vi "探头窗口-32-4列.vi"() -> ()   [LabVIEW 2017]
panel:
  in  "更新数据":T1
  in  "停止信号":bool=TRUE
  out "更新数据？":bool=TRUE
  out "引用-切回列表模式？":refnum<vi>
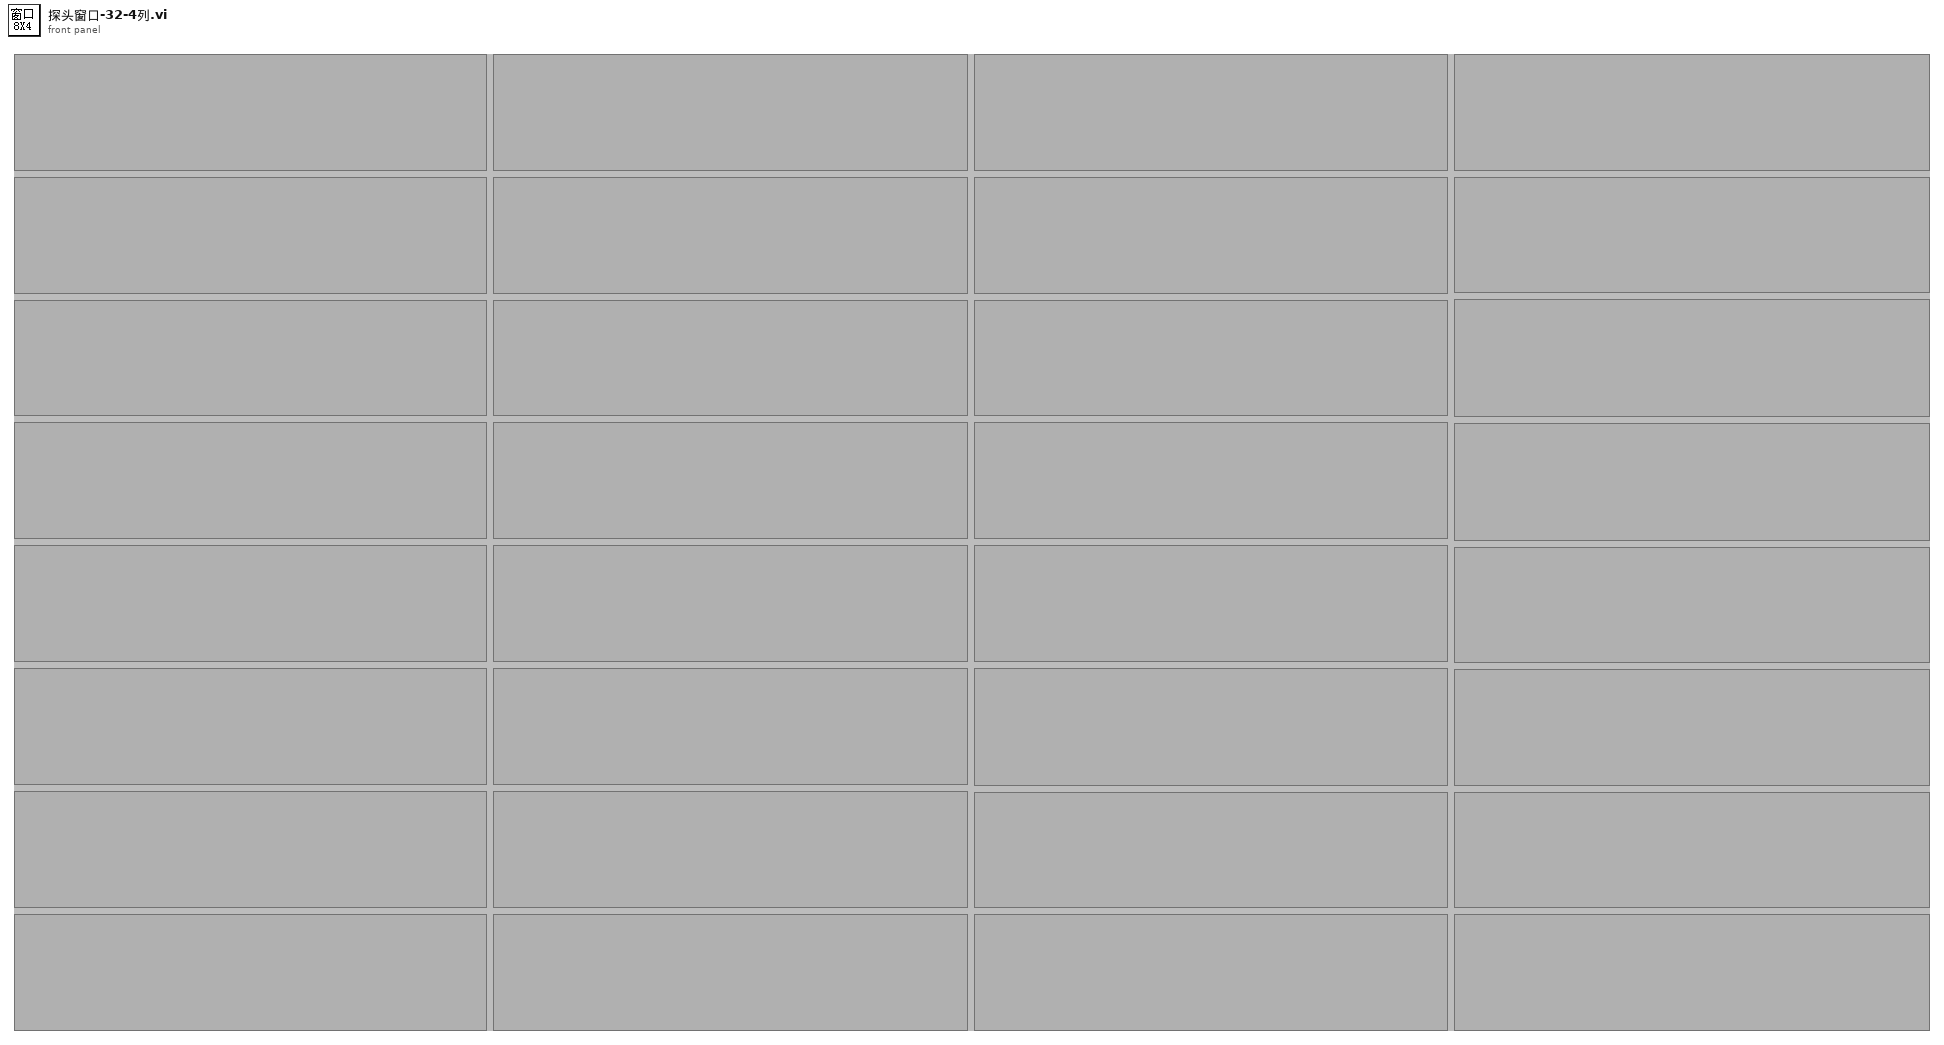
[diagram p1: front panel]
types:
  T1 = cluster{"探头启用状态？":bool[], "测量值":cluster{"X":timestamp, "Y":dbl}[], "限值":cluster{"限值1":dbl, "限值2":dbl, "探头限值":enum16{"一级限值", "二级限值"}}[], "报警状态":enum16{"正常", "一级报警", "二级报警", "累积报警"}[], "探头信息":string[], "累积剂量":cluster{"设备名称":string, "启用累积？":bool, "起始时间":timestamp, "累积剂量":dbl, "累积报警阈值":dbl}[]}
  T2 = cluster{"启用状态？":bool, "测量值":cluster{"X":timestamp, "Y":dbl}, "限值簇":cluster{"限值1":dbl, "限值2":dbl, "探头限值":enum16{"一级限值", "二级限值"}}, "报警状态":enum16{"正常", "一级报警", "二级报警", "累积报警"}, "探头信息":string, "探头地址":i32, "累积剂量":cluster{"设备名称":string, "启用累积？":bool, "起始时间":timestamp, "累积剂量":dbl, "累积报警阈值":dbl}}
  T3 = typedef "eventvkey.ctl" = enum16{"ASCII", "Enter", "Return", "Shift", "Ctrl", "Alt", "Cmd", "Opt", "Caps", "NumLock", "Clear", "Break", "Up", "Down", "Left", "Right", "Insert", "Delete", "Home", "End", "PageUp", "PageDown", "Escape", "Help", "Pause", "ScrollLock", "F1", "F2", "F3", "F4", "F5", "F6", "F7", "F8", "F9", "F10", "F11", "F12", "F13", "F14", "F15", "F16", "F17", "F18", "F19", "F20", "F21", "F22", "F23", "F24", "Play", "VolumeUp", "VolumeDown", "Mute", "Two Byte Char"}
  T4 = cluster{"限值1":dbl, "限值2":dbl, "探头限值":enum16{"一级限值", "二级限值"}}
  T5 = cluster{"限值1":dbl, "限值2":dbl, "探头限值":enum16{"一级限值", "二级限值"}}[]
  T6 = cluster{"设备名称":string, "启用累积？":bool, "起始时间":timestamp, "累积剂量":dbl, "累积报警阈值":dbl}[]
  T7 = cluster{"设备名称":string, "启用累积？":bool, "起始时间":timestamp, "累积剂量":dbl, "累积报警阈值":dbl}
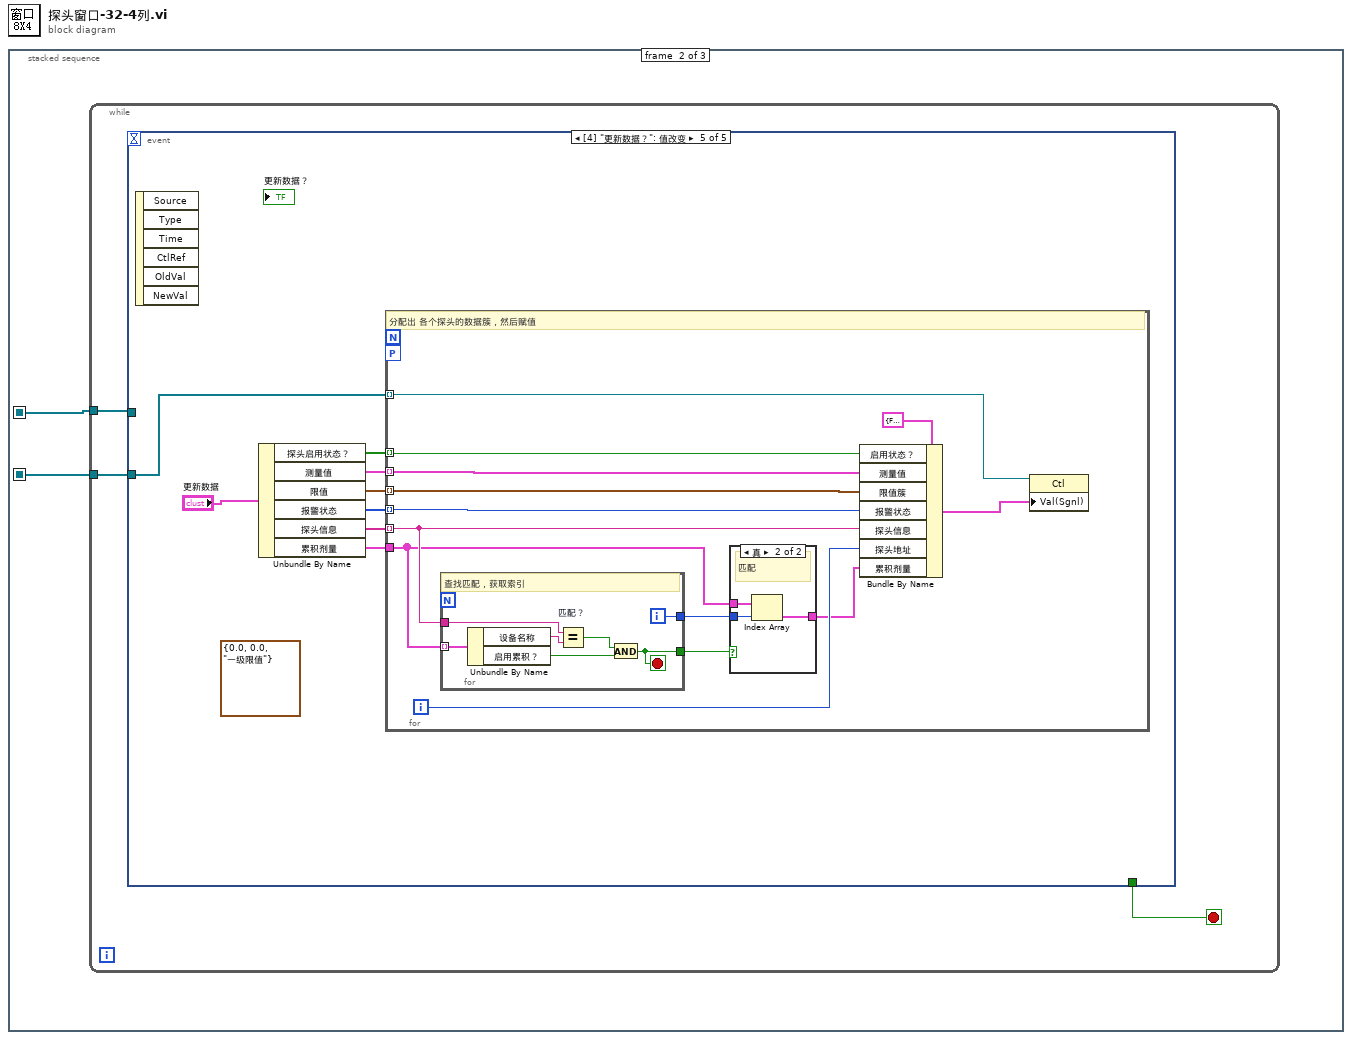
[diagram p0: block diagram]
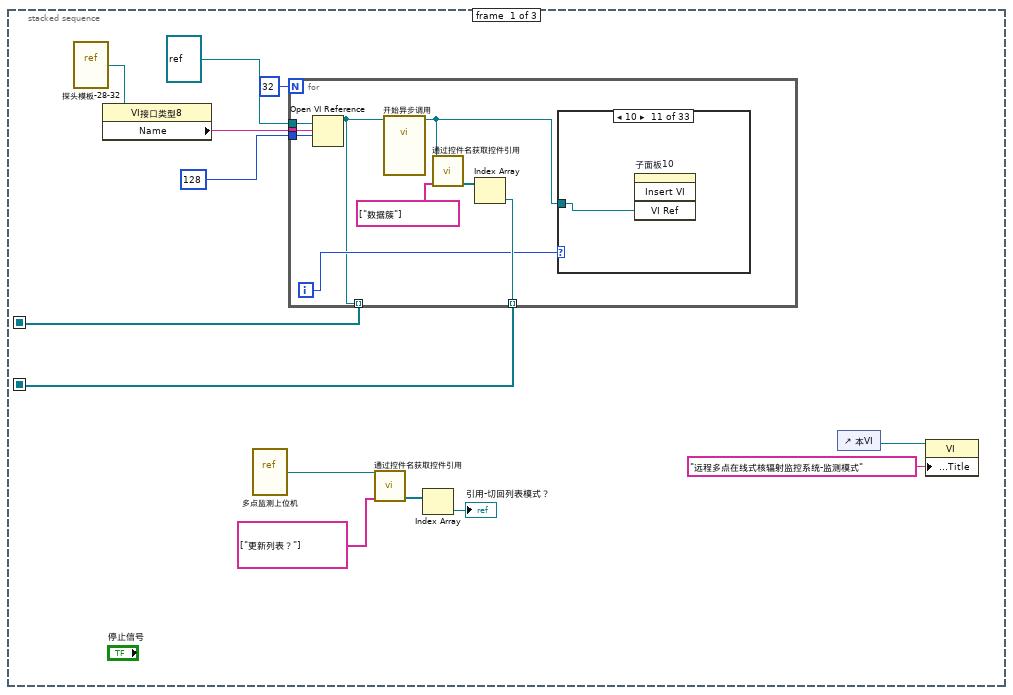
[diagram p2: hidden frame]
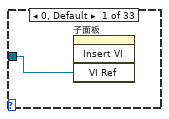
[diagram p3: hidden frame]
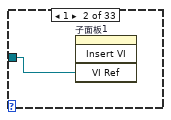
[diagram p4: hidden frame]
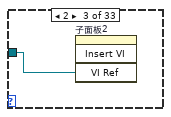
[diagram p5: hidden frame]
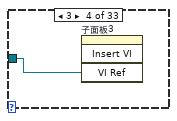
[diagram p6: hidden frame]
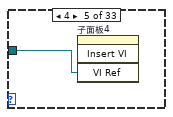
[diagram p7: hidden frame]
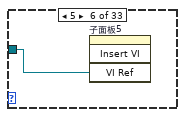
[diagram p8: hidden frame]
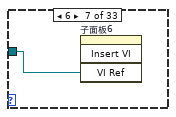
[diagram p9: hidden frame]
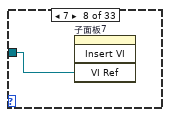
[diagram p10: hidden frame]
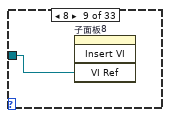
[diagram p11: hidden frame]
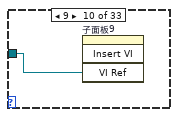
[diagram p12: hidden frame]
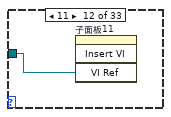
[diagram p13: hidden frame]
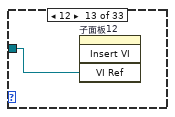
[diagram p14: hidden frame]
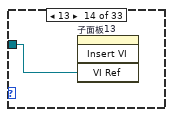
[diagram p15: hidden frame]
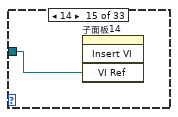
[diagram p16: hidden frame]
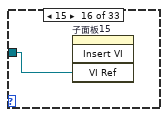
[diagram p17: hidden frame]
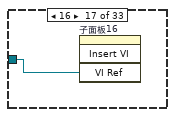
[diagram p18: hidden frame]
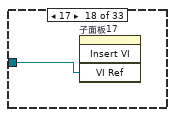
[diagram p19: hidden frame]
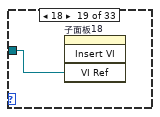
[diagram p20: hidden frame]
diagram:
  n1 = stacked-sequence {
    seq-local: [w8 _ _] -> [_ w56 _]
    seq-local: [w7 _ _] -> [_ w55 _]
    frame #0 {
      n2 = vi-ref "探头模板-28-32.vi"() -> (w13:refnum<vi>)
      n3 = property class="VI接口类型8"(reference=w13) -> ("Name"=w12:string)  [unwired: 1 in, 2 out]
      n4 = vi-ref "多点监测上位机.vi"() -> (w6:refnum<vi>)
      n5 = for {
        N: 32 -> [_]
        tunnel: w12 -> [w22]
        tunnel: 128 ("选项") -> [w21]
        tunnel: refnum<vi> refnum ("类型说明符VI引用句柄（仅用于类型）") -> [w20]
        tunnel: [w15] -> w8 mode=indexing
        tunnel: [w17] -> w7 mode=indexing
        i -> [w16]
        n6 = Open VI Reference(type specifier VI Refnum (for type only)=w20, vi path=w22, options=w21) -> (vi reference=w15:refnum<vi>)  [unwired: 3 in, 1 out]
        n7 = call-by-ref "开始异步调用"(reference=w15) -> (reference out=w14:refnum<vi>)  [unwired: 13 in, 1 out]
        n8 = call "通过控件名获取控件引用.vi"("控件名数组"=string[] ["数据簇"], "VI引用"=w14) -> ("控件引用输出"=w18:refnum<vi>[])  [unwired: 7 in, 2 out]
        n9 = Index Array(array=w18) -> (element=w17:refnum<vi>)  [unwired: 1 in]
        n10 = case shown="10" w16 {
          tunnel: w14 -> [w23 w24 w25 w26 w27 w28 w29 w30 w31 w32 w33 w34 w35 w36 w37 w38 w39 w40 w41 w42 w43 w44 w45 w46 w47 w48 w49 w50 w51 w52 w53 w54 _]
          frame 0, Default {
            n11 = invoke on="子面板" class="子面板" method="Insert VI"("VI Ref"=w23) -> ()  [unwired: 3 in, 4 out]
          }
          frame 1 {
            n12 = invoke on="子面板1" class="SubPnl" method="Insert VI"("VI Ref"=w24) -> ()  [unwired: 3 in, 4 out]
          }
          frame 2 {
            n13 = invoke on="子面板2" class="SubPnl" method="Insert VI"("VI Ref"=w25) -> ()  [unwired: 3 in, 4 out]
          }
          frame 3 {
            n14 = invoke on="子面板3" class="SubPnl" method="Insert VI"("VI Ref"=w26) -> ()  [unwired: 3 in, 4 out]
          }
          frame 4 {
            n15 = invoke on="子面板4" class="SubPnl" method="Insert VI"("VI Ref"=w27) -> ()  [unwired: 3 in, 4 out]
          }
          frame 5 {
            n16 = invoke on="子面板5" class="SubPnl" method="Insert VI"("VI Ref"=w28) -> ()  [unwired: 3 in, 4 out]
          }
          frame 6 {
            n17 = invoke on="子面板6" class="SubPnl" method="Insert VI"("VI Ref"=w29) -> ()  [unwired: 3 in, 4 out]
          }
          frame 7 {
            n18 = invoke on="子面板7" class="SubPnl" method="Insert VI"("VI Ref"=w30) -> ()  [unwired: 3 in, 4 out]
          }
          frame 8 {
            n19 = invoke on="子面板8" class="SubPnl" method="Insert VI"("VI Ref"=w31) -> ()  [unwired: 3 in, 4 out]
          }
          frame 9 {
            n20 = invoke on="子面板9" class="SubPnl" method="Insert VI"("VI Ref"=w32) -> ()  [unwired: 3 in, 4 out]
          }
          frame 10 {
            n21 = invoke on="子面板10" class="SubPnl" method="Insert VI"("VI Ref"=w33) -> ()  [unwired: 3 in, 4 out]
          }
          frame 11 {
            n22 = invoke on="子面板11" class="SubPnl" method="Insert VI"("VI Ref"=w34) -> ()  [unwired: 3 in, 4 out]
          }
          frame 12 {
            n23 = invoke on="子面板12" class="SubPnl" method="Insert VI"("VI Ref"=w35) -> ()  [unwired: 3 in, 4 out]
          }
          frame 13 {
            n24 = invoke on="子面板13" class="SubPnl" method="Insert VI"("VI Ref"=w36) -> ()  [unwired: 3 in, 4 out]
          }
          frame 14 {
            n25 = invoke on="子面板14" class="SubPnl" method="Insert VI"("VI Ref"=w37) -> ()  [unwired: 3 in, 4 out]
          }
          frame 15 {
            n26 = invoke on="子面板15" class="SubPnl" method="Insert VI"("VI Ref"=w38) -> ()  [unwired: 3 in, 4 out]
          }
          frame 16 {
            n27 = invoke on="子面板16" class="SubPnl" method="Insert VI"("VI Ref"=w39) -> ()  [unwired: 3 in, 4 out]
          }
          frame 17 {
            n28 = invoke on="子面板17" class="SubPnl" method="Insert VI"("VI Ref"=w40) -> ()  [unwired: 3 in, 4 out]
          }
          frame 18 {
            n29 = invoke on="子面板18" class="SubPnl" method="Insert VI"("VI Ref"=w41) -> ()  [unwired: 3 in, 4 out]
          }
          frame 19 {
            n30 = invoke on="子面板19" class="SubPnl" method="Insert VI"("VI Ref"=w42) -> ()  [unwired: 3 in, 4 out]
          }
          frame 20 {
            n31 = invoke on="子面板20" class="SubPnl" method="Insert VI"("VI Ref"=w43) -> ()  [unwired: 3 in, 4 out]
          }
          frame 21 {
            n32 = invoke on="子面板21" class="SubPnl" method="Insert VI"("VI Ref"=w44) -> ()  [unwired: 3 in, 4 out]
          }
          frame 22 {
            n33 = invoke on="子面板22" class="SubPnl" method="Insert VI"("VI Ref"=w45) -> ()  [unwired: 3 in, 4 out]
          }
          frame 23 {
            n34 = invoke on="子面板23" class="SubPnl" method="Insert VI"("VI Ref"=w46) -> ()  [unwired: 3 in, 4 out]
          }
          frame 24 {
            n35 = invoke on="子面板24" class="SubPnl" method="Insert VI"("VI Ref"=w47) -> ()  [unwired: 3 in, 4 out]
          }
          frame 25 {
            n36 = invoke on="子面板25" class="SubPnl" method="Insert VI"("VI Ref"=w48) -> ()  [unwired: 3 in, 4 out]
          }
          frame 26 {
            n37 = invoke on="子面板26" class="SubPnl" method="Insert VI"("VI Ref"=w49) -> ()  [unwired: 3 in, 4 out]
          }
          frame 27 {
            n38 = invoke on="子面板27" class="SubPnl" method="Insert VI"("VI Ref"=w50) -> ()  [unwired: 3 in, 4 out]
          }
          frame 28 {
            n39 = invoke on="子面板28" class="SubPnl" method="Insert VI"("VI Ref"=w51) -> ()  [unwired: 3 in, 4 out]
          }
          frame 29 {
            n40 = invoke on="子面板29" class="SubPnl" method="Insert VI"("VI Ref"=w52) -> ()  [unwired: 3 in, 4 out]
          }
          frame 30 {
            n41 = invoke on="子面板30" class="SubPnl" method="Insert VI"("VI Ref"=w53) -> ()  [unwired: 3 in, 4 out]
          }
          frame 31 {
            n42 = invoke on="子面板31" class="SubPnl" method="Insert VI"("VI Ref"=w54) -> ()  [unwired: 3 in, 4 out]
          }
          frame 32 {
          }
        }
      }
      n43 = call "通过控件名获取控件引用.vi"("控件名数组"=string[] ["更新列表？"], "VI引用"=w6) -> ("控件引用输出"=w4:refnum<vi>[])  [unwired: 7 in, 2 out]
      n44 = Index Array(array=w4) -> (element=→"引用-切回列表模式？":refnum<vi>)  [unwired: 1 in]
      n45 = control-ref of="本VI"() -> (w2:refnum<vi>)
      n46 = property class="VI"(reference=w2, "Front Panel.Title"="远程多点在线式核辐射监控系统-监测模式" ("前面板窗口:标题")) -> ()  [unwired: 1 in, 2 out]
    }
    frame #1 {
      n47 = while {
        tunnel: w56 -> [w58]
        tunnel: w55 -> [w57]
        stop <- w59 stop-if-true
        n48 = event shown="[4] \"更新数据？\": 值改变" {
          selector: _ -> [_ _ _ _ _]
          dyn-events: _ -> [_ _ _ _ _]
          timeout: _ -> [_ _ _ _ _]
          tunnel: [_ TRUE ("放弃？") _ _ _] -> w59
          tunnel: w58 -> [_ w63 _ _ _]
          tunnel: w57 -> [_ _ _ _ w71]
          event Timeout {
            n49 = event-data() -> ()  [unwired: 1 in, 3 out]
          }
          event "停止信号": Value Change {
            w62 = TRUE  # T
            n50 = event-data() -> ()  [unwired: 1 in, 6 out]
            n51 = for {
              tunnel: w63 -> [w67] mode=indexing
              n52 = invoke class="VI (严格)" method="Abort VI"(reference=w67) -> (reference out=w65:refnum<vi>, error out=w66:errorcluster)  [unwired: 2 in, 1 out]
              n53 = Close Reference(reference=w65, error in (no error)=w66) -> (error out=w64:errorcluster)
              n54 = call <vilib>:"Clear Errors.vi"("error in (no error)"=w64) -> ()  [unwired: 5 in, 2 out]
            }
            n55 = local read "引用-切回列表模式？"() -> (w61:refnum<vi>)
            n56 = property class="Ctl"(reference=w61, "Val(Sgnl)"=w62) -> ()  [unwired: 1 in, 2 out]
          }
          event Panel Close? {
            n57 = event-data() -> ()  [unwired: 1 in, 4 out]
            n58 = property on="停止信号" class="Bool (严格)"("Val(Sgnl)"=FALSE ("值(信号)")) -> ()  [unwired: 2 in, 2 out]
            n59 = event-data() -> ()  [unwired: 2 in, 1 out]
          }
          event Key Down {
            n60 = event-data() -> ("VKey"=w69:T3)  [unwired: 1 in, 9 out]
            n61 = case shown="\"Enter\"" w69 {
              frame "ASCII", Default {
              }
              frame "Enter" {
                w70 = TRUE  # T
                n62 = property on="停止信号" class="Bool (严格)"("Val(Sgnl)"=w70) -> ()  [unwired: 2 in, 2 out]
              }
            }
          }
          event "更新数据？": Value Change {
            (unwired) T4 {"限值1"=0.0, "限值2"=0.0, "探头限值"=enum."一级限值"} ("探头限值簇")
            n63 = event-data() -> ()  [unwired: 1 in, 6 out]
            n64 = Unbundle By Name("更新数据") -> ("探头启用状态？"=w72:bool[], "测量值"=w73:cluster{"X":timestamp, "Y":dbl}[], "限值"=w74:T5, "报警状态"=w75:enum16{"正常", "一级报警", "二级报警", "累积报警"}[], "探头信息"=w76:string[], "累积剂量"=w77:T6)
            n65 = for {
              tunnel: w72 -> [w91] mode=indexing
              tunnel: w73 -> [w90] mode=indexing
              tunnel: w74 -> [w89] mode=indexing
              tunnel: w75 -> [w88] mode=indexing
              tunnel: w76 -> [w83] mode=indexing
              workers-P: _ -> [_]
              tunnel: w71 -> [w86] mode=indexing
              tunnel: w77 -> [w82]
              i -> [w84]
              # "分配出 各个探头的数据簇，然后赋值"
              n66 = for {
                tunnel: w82 -> [w101] mode=indexing
                tunnel: w83 -> [w99]
                tunnel: [w96] -> w81
                tunnel: [w95] -> w80
                i -> [w96]
                stop <- w95 stop-if-true
                # "查找匹配，获取索引"
                n67 = Unbundle By Name(w101) -> ("设备名称"=w100:string, "启用累积？"=w97:bool)
                n68 = Equal? "匹配？"(x=w99, y=w100) -> (x = y?=w98:bool)
                n69 = And(x=w98, y=w97) -> (x .and. y?=w95:bool)
              }
              n70 = case shown="真" w80 {
                tunnel: w82 -> [_ w94]
                tunnel: w81 -> [_ w93]
                tunnel: [_ w92] -> w79
                frame False {
                  # "不匹配"
                }
                frame True {
                  # "匹配"
                  n71 = Index Array(array=w94, index=w93) -> (element=w92:T7)
                }
              }
              n72 = Bundle By Name(cluster=T2 {"启用状态？"=FALSE, "测量值"={"X"=timestamp(0 s since 1904-01-01), "Y"=0.0}, "限值簇"={"限值1"=0.0, "限值2"=0.0, "探头限值"=enum."一级限值"}, "报警状态"=enum."正常", "探头信息"="", "探头地址"=0, "累积剂量"={"设备名称"="", "启用累积？"=FALSE, "起始时间"=timestamp(0 s since 1904-01-01), "累积剂量"=0.0, "累积报警阈值"=0.0}} ("输出簇"), "启用状态？"=w91, "测量值"=w90, "限值簇"=w89, "报警状态"=w88, "探头信息"=w83, "探头地址"=w84, "累积剂量"=w79) -> (w85:T2)
              n73 = property class="Ctl"(reference=w86, "Val(Sgnl)"=w85) -> ()  [unwired: 1 in, 2 out]
            }
          }
        }
      }
    }
    frame #2 {
      n74 = control-ref of="本VI"() -> (w105:refnum<vi>)
      n75 = invoke class="VI" method="FP.Close"(reference=w105) -> (reference out=w104:refnum<vi>, error out=w103:errorcluster)  [unwired: 2 in, 1 out]
      n76 = invoke class="VI" method="Abort VI"(reference=w104, error in=w103) -> (error out=w102:errorcluster)  [unwired: 1 in, 2 out]
      n77 = call <vilib>:"Clear Errors.vi"("error in (no error)"=w102) -> ()  [unwired: 5 in, 2 out]
    }
  }
